vi "Check if Reference.vi"(8 "error in (no error)":errorcluster, 11 "motor communication in":refnum<class "NI_Robotics_Motor Communication Ref.lvclass">) -> (0 "error out":errorcluster, 1 "initialized?":bool, 2 "invalid refs?":bool, 3 "motor communication out":refnum<class "NI_Robotics_Motor Communication Ref.lvclass">)   [LabVIEW 2017, in "NI_Robotics_Motor Communication Ref.lvclass"]
uses:
  <vilib>/robotics/Actuation/Motor Communication Ref/NI_Robotics_Motor Communication Ref.lvclass
  c:/Program Files (x86)/National Instruments/LabVIEW 2017/vi.lib/robotics/Actuation/Motor Communication/NI_Robotics_Motor Communication.lvclass
  <vilib>/robotics/Actuation/Motor Communication Ref/NI_Robotics_Motor Communication Ref.lvclass/NI_Robotics_Motor Communication Ref.ctl
  <vilib>/robotics/Actuation/Motor Communication/NI_Robotics_Motor Communication.lvclass/NI_Robotics_Motor Communication.ctl
  <vilib>/robotics/Actuation/Motor Communication/NI_Robotics_Motor Communication.lvclass
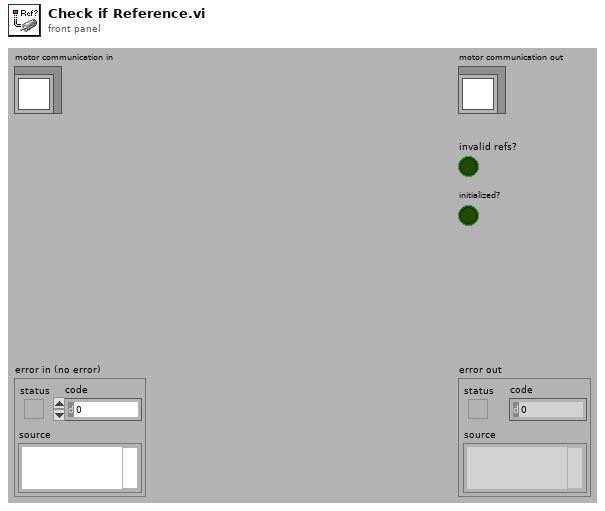
[diagram p1: front panel]
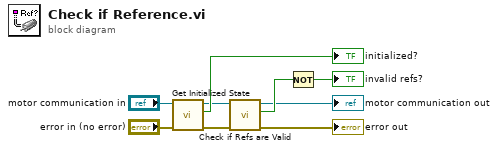
[diagram p0: block diagram]
diagram:
  n1 = call <vilib>:"Get Initialized State.vi"("error in (no error)"="error in (no error)", "motor communication in"="motor communication in") -> ("error out"=w4:errorcluster, "initialized"=→"initialized?":bool, "motor communication out"=w6:refnum<class "NI_Robotics_Motor Communication Ref.lvclass">)  [unwired: 7 in]
  n2 = call <vilib>:"Check if Refs are Valid.vi"("error in (no error)"=w4, "motor communication ref in"=w6) -> ("error out"=→"error out":errorcluster, "valid?"=w8:bool, "motor communication ref out"=→"motor communication out":refnum<class "NI_Robotics_Motor Communication Ref.lvclass">)  [unwired: 7 in]
  n3 = Not(x=w8) -> (.not. x?=→"invalid refs?":bool)
